vi "外观 2.vi"(0 "Data In":T9 caption="数据输入" {"数值" format="%04x"}, 2 "Display State In":T7 caption="显示状态输入" {"值" items=["三通阀", "排阀"]}, 3 "Container State":T8 caption="容器状态") -> (6 "Data Out":T9 caption="数据输出" {"数值" format="%04x"}, 7 "Display State Out":T7 caption="显示状态输出" {"值" items=["三通阀", "排阀"]}, 8 "Action":T6 caption="动作")   [LabVIEW 2016, in "CODMn调试控件V3.xctl"]
uses:
  <vilib>/_xctls/Container State.ctl
  <vilib>/_xctls/Action.ctl
  <vilib>/_xctls/XControlSupport.lvlib
panel:
  in  "缺液检测":bool caption="V2"
  in  "偏心轮:":u16 caption="mL"
  in  "模式":enum32{"测试模式", "流程模式"}(tab)
  in  "外设:":T1
  in  "加热:":bool caption="V2"
  in  "摄氏度":u16
  in  "量:":u16=5000
  in  "注射泵:":T2(radio)
  in  "进样:":T3(radio)
  out "阀配置":u8(ring) items=["三通阀", "排阀"]
  in  "柱塞泵体积/等待时间":u16=5000
  in  "功能选择":enum32{"等待", "复位", "注入", "注出"}(radio)=enum."注入"
  out "选项卡控件":enum32{"选项卡 1", "选项卡 2"}(tab)
  in  "阀口选择":T4(radio)
  in  "其他":enum32{"未选择", "更新A值", "更新B值", "反滴定"}(radio)
  in  "反应杯温度控制:":u16
  in  "偏心轮抽取液体次数:":u16
  in  "外设":T5
  out "字符串":string="柱塞泵体积μL"
  # "uL"
  # "℃"
  # "次(0代表不动作)"
  # "℃(0代表不控温)"
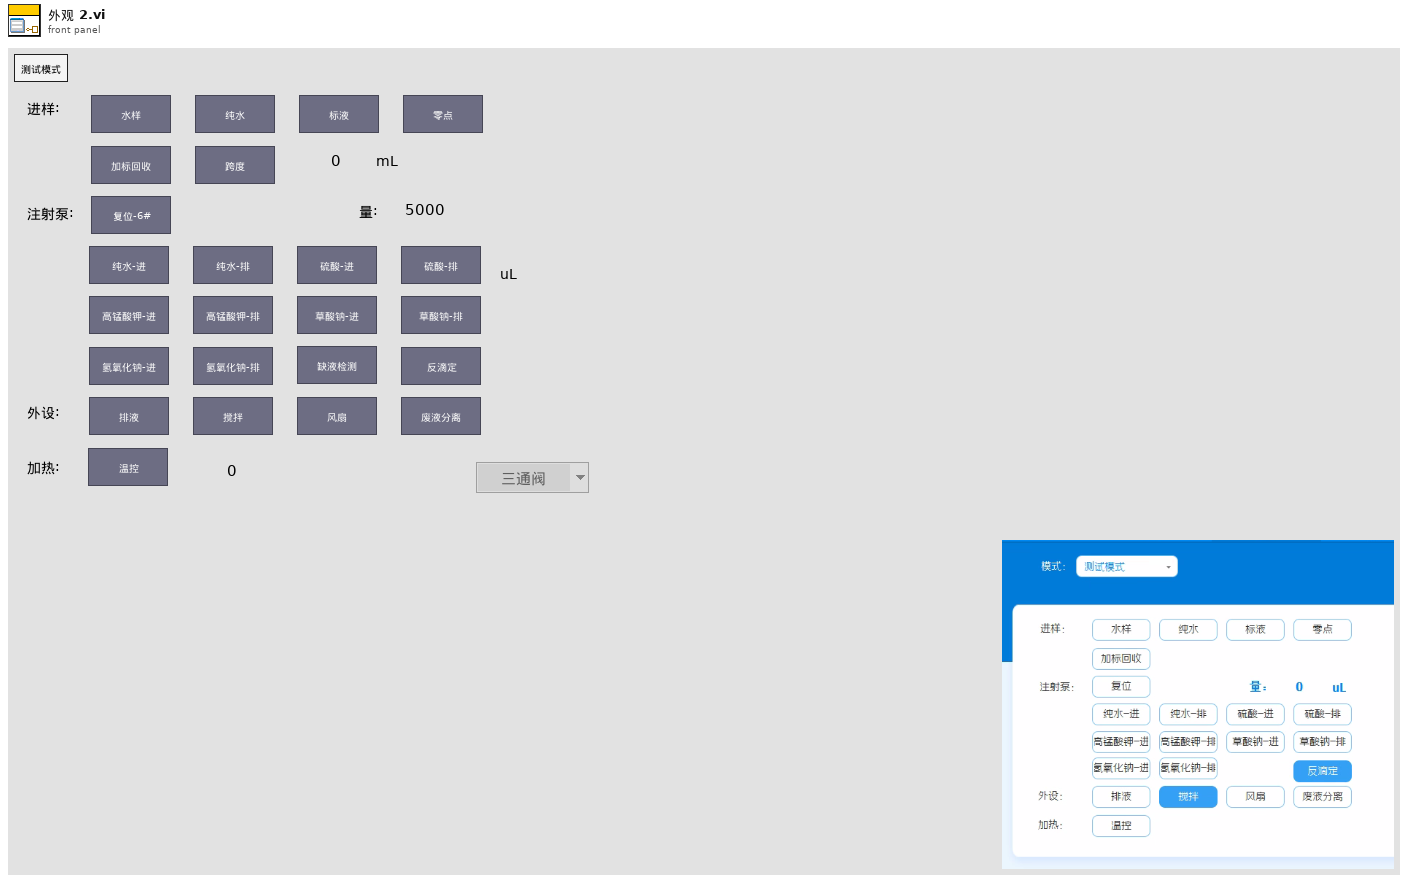
[diagram p1: front panel]
types:
  T1 = cluster{"排液":bool, "搅拌":bool, "风扇":bool, "废液分离":bool}
  T2 = enum32{"未选择", "纯水-进", "纯水-排", "硫酸-进", "硫酸-排", "复位", "高锰酸钾-进", "高锰酸钾-排", "草酸钠-进", "草酸钠-排", "氢氧化钠-进", "氢氧化钠-排", "反滴定"}
  T3 = enum32{"未选择", "水样", "纯水", "标液", "零点", "加标回收", "跨度"}
  T4 = enum32{"未选择", "V1", "V2", "V3", "V4", "V5", "V6", "V7", "V8", "V9", "V10", "V11", "V12"}
  T5 = cluster{"排液阀":bool, "搅拌":bool, "冷凝风扇":bool, "废液分离阀":bool, "电磁阀1":bool, "电磁阀2":bool, "电磁阀3":bool, "电磁阀4":bool, "电磁阀5":bool, "电磁阀6":bool}
  T6 = typedef "XControlSupport.lvlib/Action.ctl" = cluster{"Data Changed?":bool, "State Changed?":bool, "Action Name":string}
  T7 = typedef "CODMn调试控件V3.xctl/状态 2.ctl" = cluster{"值":u8}
  T8 = typedef "XControlSupport.lvlib/Container State.ctl" = cluster{"Indicator?":bool, "Run Mode?":bool, " Refnum":refnum<vi>}
  T9 = typedef "CODMn调试控件V3.xctl/数据 2.ctl" = cluster{"数值":u16[], "模式":enum32{"测试模式", "流程模式"}}
  T10 = enum32{"未选择", "水样", "纯水", "标液", "零点", "加标回收", "加标回收 2"}
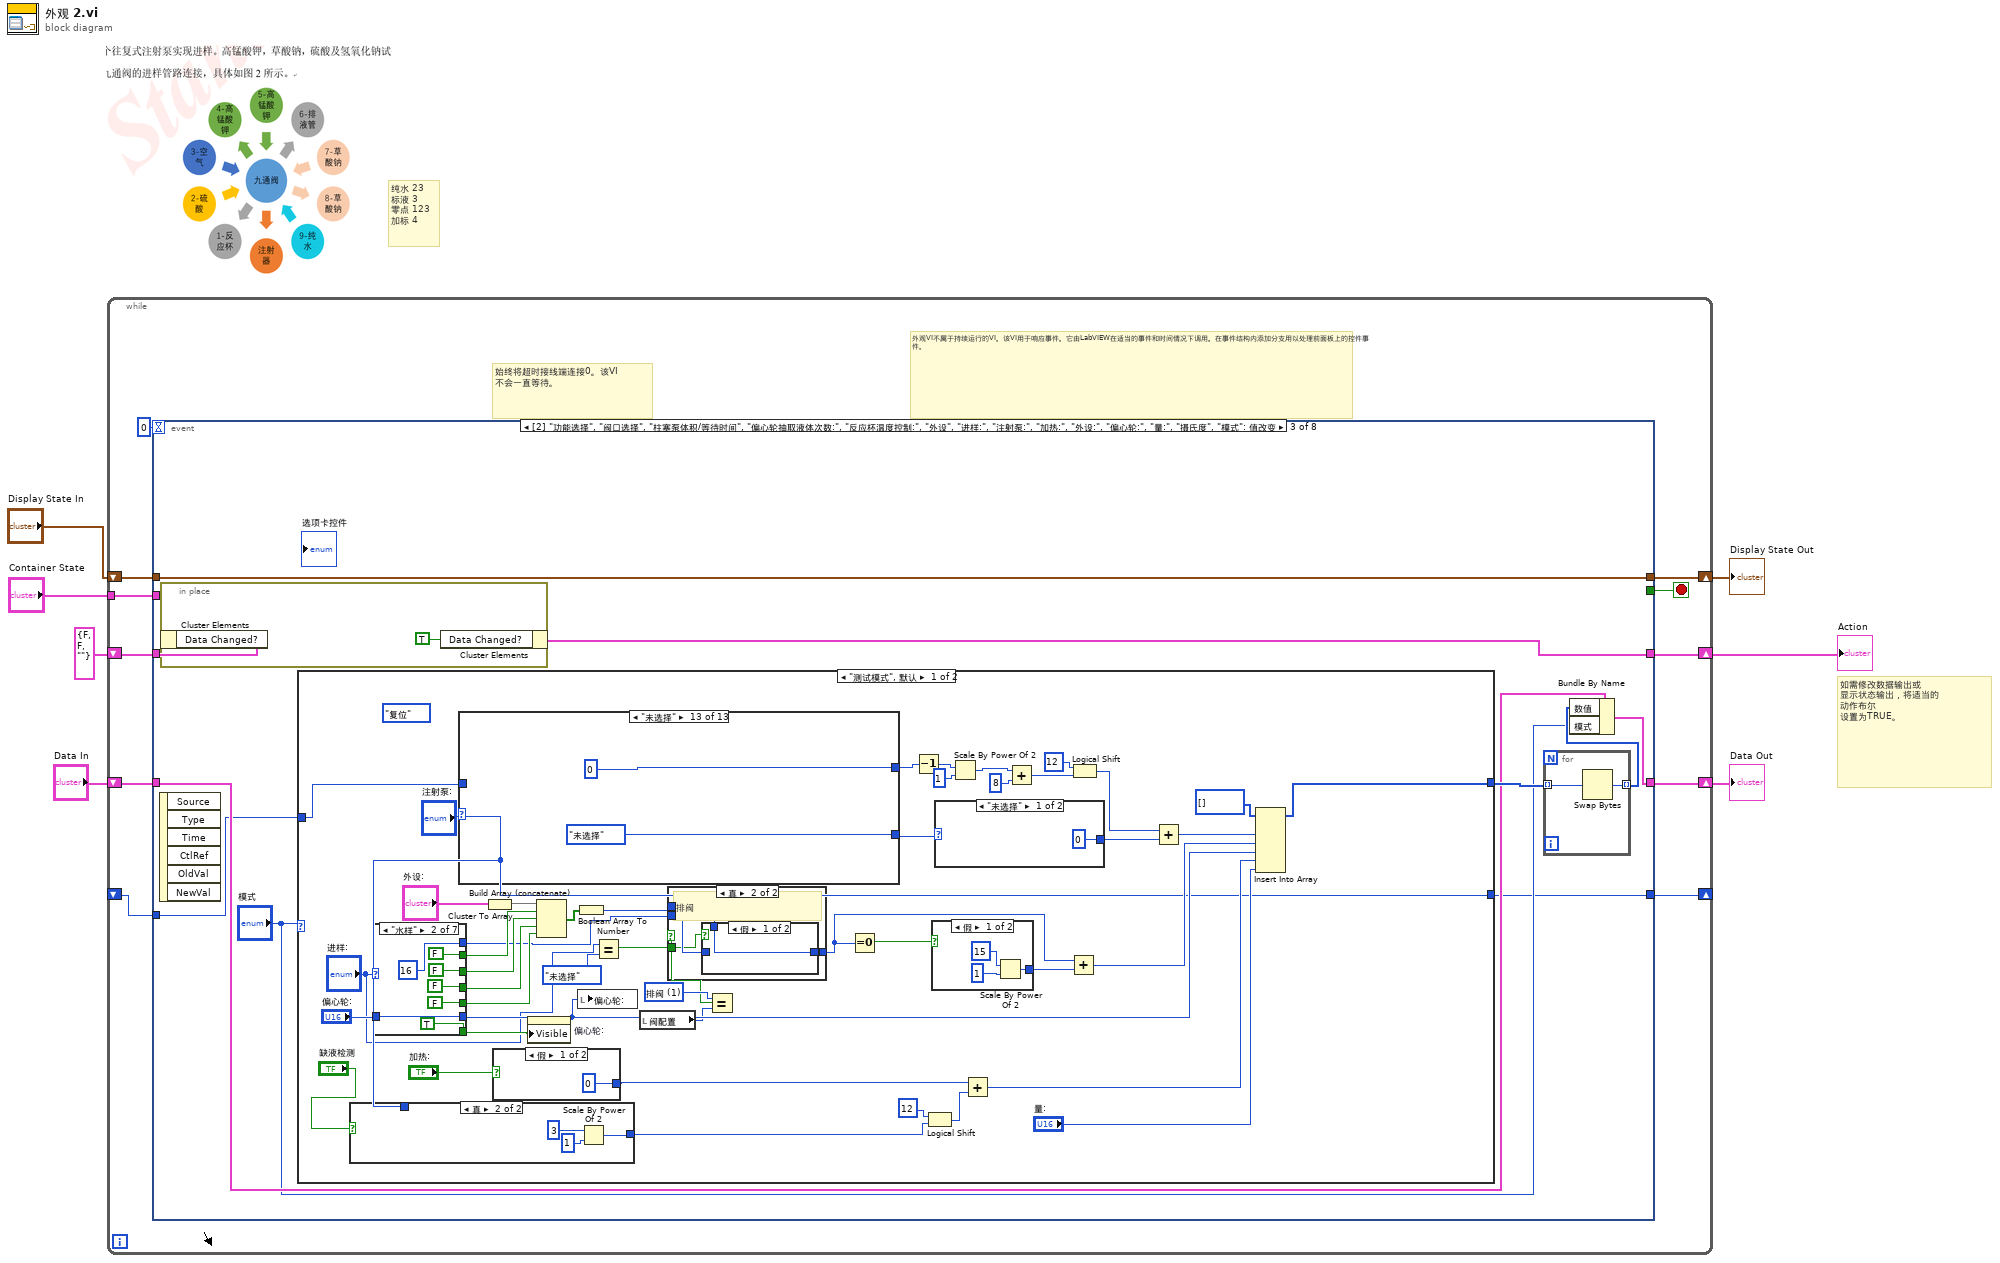
[diagram p0: block diagram]
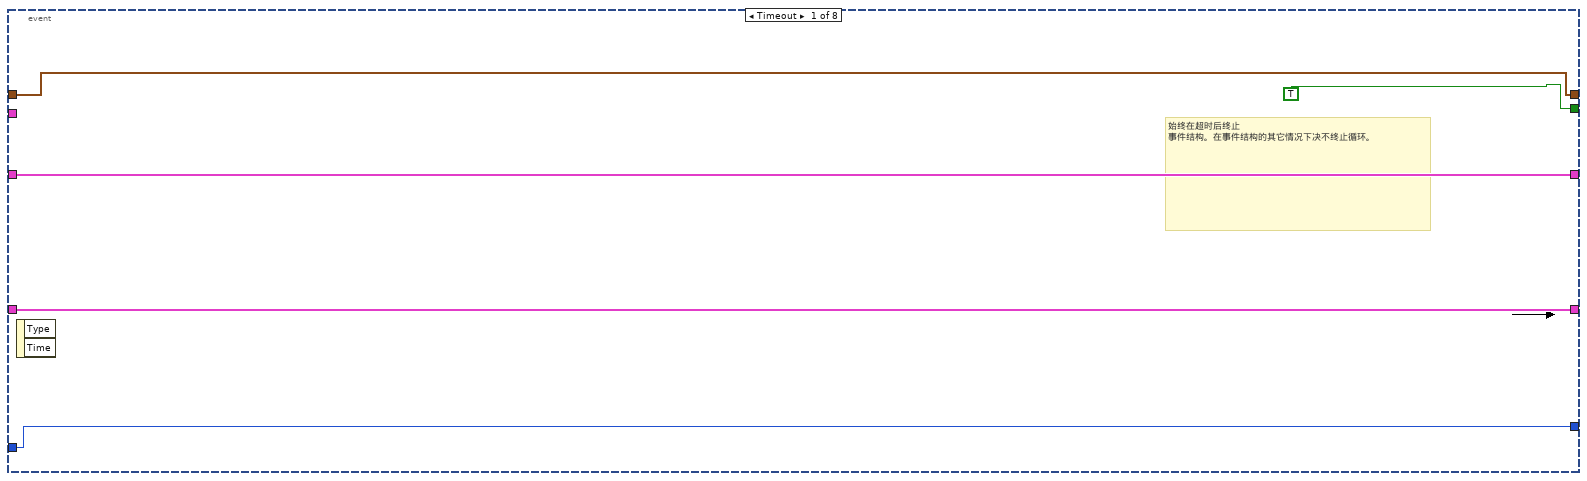
[diagram p2: hidden frame]
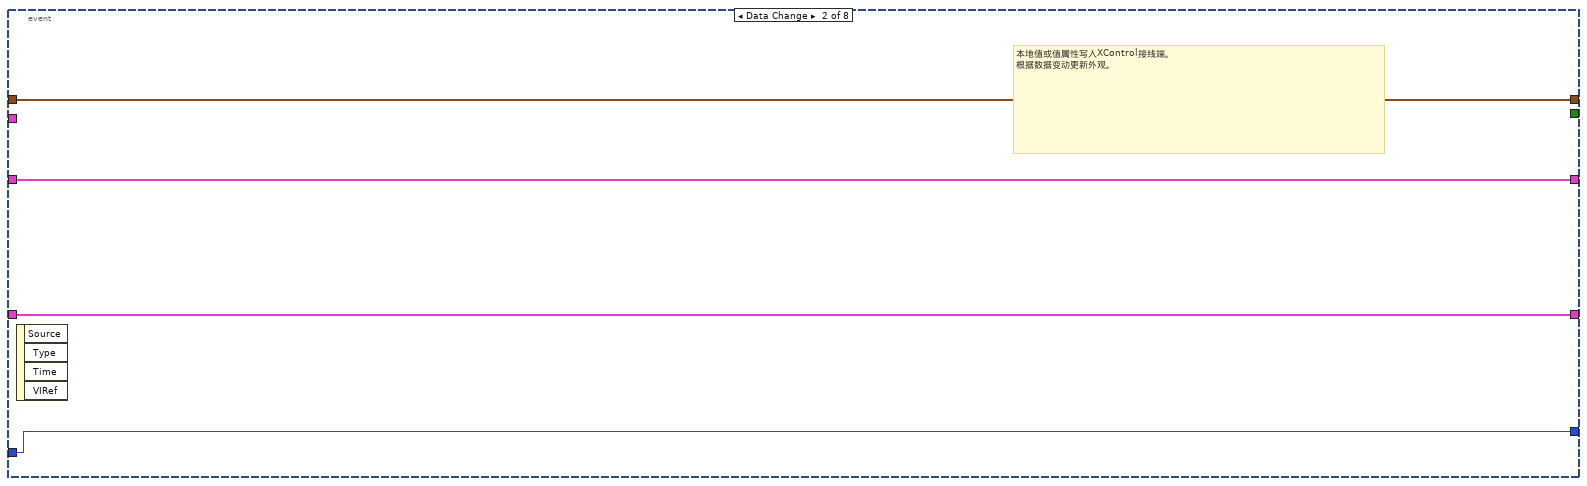
[diagram p3: hidden frame]
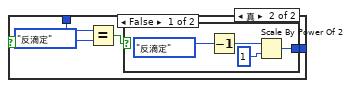
[diagram p6: hidden frame]
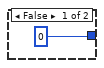
[diagram p7: hidden frame]
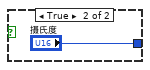
[diagram p8: hidden frame]
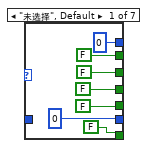
[diagram p9: hidden frame]
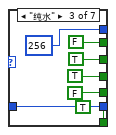
[diagram p10: hidden frame]
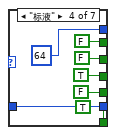
[diagram p11: hidden frame]
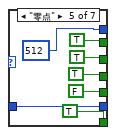
[diagram p12: hidden frame]
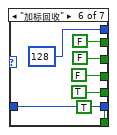
[diagram p13: hidden frame]
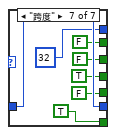
[diagram p14: hidden frame]
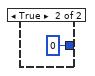
[diagram p15: hidden frame]
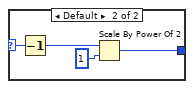
[diagram p16: hidden frame]
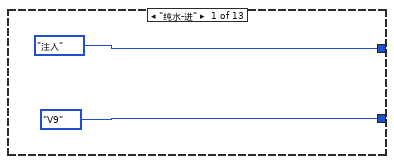
[diagram p17: hidden frame]
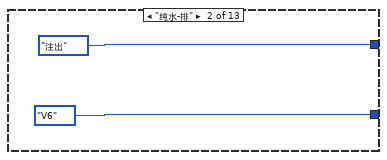
[diagram p18: hidden frame]
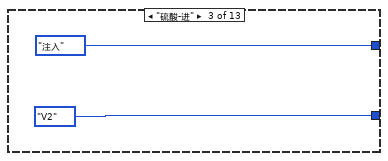
[diagram p19: hidden frame]
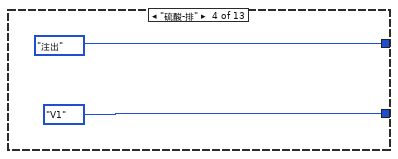
[diagram p20: hidden frame]
diagram:
  # "纯水 23\n标液 3\n零点 123\n加标 4"
  # "如需修改数据输出或\n显示状态输出，将适当的\n动作布尔\n设置为TRUE。"
  n1 = while {
    shift-right: [w17] -> w4
    shift-left: "Display State In" -> [w18]
    tunnel: "Container State" -> [w14]
    shift-right: [w12] -> w7
    shift-left: "Data In" -> [w13]
    shift-right: [w10] -> w2
    shift-left: T6 {"Data Changed?"=FALSE, "State Changed?"=FALSE, "Action Name"=""} ("Action") -> [w11]
    shift-right: [w9] -> _
    shift-left: _ -> [w8]
    stop <- w16 stop-if-true
    # "外观VI不属于持续运行的VI。该VI用于响应事件。它由LabVIEW在适当的事件和时间情况下调用。在事件结构内添加分支用以处理前面板上的控件事件。"
    # "始终将超时接线端连接0。该VI\n不会一直等待。"
    n2 = event shown="[2] \"功能选择\", \"阀口选择\", \"柱塞泵体积/等待时间\", \"偏心轮抽取液体次数:\", \"反应杯温度控制:\", \"外设\", \"进样:\", \"注射泵:\", \"加热:\", \"外设:\", \"偏心轮:\", \"量:\", \"摄氏度\", \"模式\": 值改变" {
      selector: _ -> [_ _ _ _ _ _ _ _]
      dyn-events: _ -> [_ _ _ _ _ _ _ _]
      timeout: 0 -> [_ _ _ _ _ _ _ _]
      tunnel: w18 -> [w21 w24 w37 w305 w317 w318 w326 w330]
      tunnel: [w21 w24 w37 w305 w317 w318 w326 w330] -> w17
      tunnel: [TRUE _ _ _ _ _ _ _] -> w16
      tunnel: w14 -> [_ _ _ _ _ _ w327 w332]
      tunnel: w13 -> [w20 w27 w33 w304 w316 w322 w325 w329]
      tunnel: [w20 w27 w30 w304 w316 w322 w325 w329] -> w12
      tunnel: [w22 w26 w35 w303 w315 w321 w324 w328] -> w10
      tunnel: w11 -> [w22 w26 w36 w303 w315 w321 w324 w328]
      tunnel: [w19 w25 w29 w298 w310 w320 w323 w331] -> w9
      tunnel: w8 -> [w19 w25 w28 w298 w310 w320 w323 w331]
      event Timeout {
        # "始终在超时后终止\n事件结构。在事件结构的其它情况下决不终止循环。"
        n3 = event-data() -> ()  [unwired: 1 in, 2 out]
      }
      event Data Change {
        # "本地值或值属性写入XControl接线端。\n根据数据变动更新外观。"
        n4 = event-data() -> ()  [unwired: 1 in, 4 out]
      }
      event "功能选择", "阀口选择", "柱塞泵体积/等待时间", "偏心轮抽取液体次数:", "反应杯温度控制:", "外设", "进样:", "注射泵:", "加热:", "外设:", "偏心轮:", "量:", "摄氏度", "模式": Value Change {
        n5 = event-data() -> ()  [unwired: 1 in, 6 out]
        n6 = in-place {
          n7 = in-place-cluster #1(w36) -> ()  [unwired: 1 out]
          n8 = in-place-cluster #1("Data Changed?"=TRUE) -> (w35:T6)
        }
        n9 = case shown="\"测试模式\", 默认" "模式" {
          tunnel: [w60 w249] -> w34
          tunnel: ["注射泵:" w242] -> w29
          tunnel: w28 -> [w47 w242]
          frame "测试模式", Default {
            w41 = u8 1 items=["三通阀", "排阀"] ("Value")
            (unwired) enum32{"等待", "复位", "注入", "注出"}."复位" ("功能选择")
            n10 = case shown="真" "缺液检测" {
              tunnel: "注射泵:" -> [w92 _]
              tunnel: [w90 w100] -> w62
              frame False {
                n11 = Equal?(x=w92, y=T2."反滴定" ("注射泵:")) -> (x = y?=w91:bool)
                n12 = case shown="真" w91 {
                  tunnel: [i16 0 w95] -> w90
                  frame False {
                  }
                  frame True {
                    n13 = Decrement(x=enum32{"未选择", "更新A值", "更新B值", "反滴定"}."反滴定" ("其他")) -> (x-1=w96:enum32{"未选择", "更新A值", "更新B值", "反滴定"})
                    n14 = Scale By Power Of 2(n=w96, x=i16 1 ("y")) -> (x*2^n=w95:i16)
                  }
                }
              }
              frame True {
                n15 = Scale By Power Of 2(n=i16 3, x=i16 1 ("y")) -> (x*2^n=w100:i16)
              }
            }
            n16 = case shown="\"水样\"" "进样:" {
              tunnel: [FALSE FALSE FALSE FALSE TRUE FALSE FALSE] -> w74
              tunnel: [FALSE FALSE TRUE FALSE TRUE FALSE FALSE] -> w73
              tunnel: [FALSE FALSE TRUE TRUE TRUE FALSE TRUE] -> w72
              tunnel: [FALSE FALSE FALSE FALSE FALSE TRUE FALSE] -> w71
              tunnel: "偏心轮:" -> [_ w113 w120 w127 w134 w141 w151]
              tunnel: [u16 0 ("偏心轮:") w113 w120 w127 w134 w141 w151] -> w57
              tunnel: [FALSE TRUE TRUE TRUE TRUE TRUE TRUE] -> w56
              tunnel: [u16 0 ("数字") u16 16 ("数字") u16 256 ("数字") u16 64 ("数字") u16 512 ("数字") u16 128 ("数字") u16 32 ("数字")] -> w42
              frame "未选择", Default {
              }
              frame "水样" {
              }
              frame "纯水" {
              }
              frame "标液" {
              }
              frame "零点" {
              }
              frame "加标回收" {
              }
              frame "跨度" {
              }
            }
            n17 = case shown="\"未选择\"" "注射泵:" {
              tunnel: [enum32{"等待", "复位", "注入", "注出"}."注入" ("功能选择") enum32{"等待", "复位", "注入", "注出"}."注出" ("功能选择") enum32{"等待", "复位", "注入", "注出"}."注入" ("功能选择") enum32{"等待", "复位", "注入", "注出"}."注出" ("功能选择") enum32{"等待", "复位", "注入", "注出"}."复位" ("功能选择") enum32{"等待", "复位", "注入", "注出"}."注入" ("功能选择") enum32{"等待", "复位", "注入", "注出"}."注出" ("功能选择") enum32{"等待", "复位", "注入", "注出"}."注入" ("功能选择") enum32{"等待", "复位", "注入", "注出"}."注出" ("功能选择") enum32{"等待", "复位", "注入", "注出"}."注入" ("功能选择") enum32{"等待", "复位", "注入", "注出"}."注出" ("功能选择") 0 0] -> w59
              tunnel: [T4."V9" ("阀口选择") T4."V6" ("阀口选择") T4."V2" ("阀口选择") T4."V1" ("阀口选择") T4."V6" ("阀口选择") T4."V5" ("阀口选择") T4."V4" ("阀口选择") T4."V7" ("阀口选择") T4."V8" ("阀口选择") T4."V3" ("阀口选择") T4."V6" ("阀口选择") T4."未选择" ("阀口选择") T4."未选择" ("阀口选择")] -> w80
              tunnel: w47 -> [_ _ _ _ _ w172 w181 w190 w205 w220 w229 _ _]
              frame "纯水-进" {
              }
              frame "纯水-排" {
              }
              frame "硫酸-进" {
              }
              frame "硫酸-排" {
              }
              frame "复位" {
              }
              frame "高锰酸钾-进" {
                n18 = Greater Or Equal?(x=w172, y=T2."草酸钠-进" ("注射泵:")) -> (x >= y?=w175:bool)
                n19 = Less Or Equal?(x=w172, y=T2."氢氧化钠-排" ("注射泵:")) -> (x <= y?=w176:bool)
                n20 = And(x=w175, y=w176) -> (x .and. y?=w177:bool)
                n21 = case shown="真" w177 {
                  frame False {
                  }
                  frame True {
                    n22 = One Button Dialog(message="“\"警告:未进行润洗\n或者进出液不匹配\"”" ("消息")) -> ()  [unwired: 1 in, 1 out]
                  }
                }
              }
              frame "高锰酸钾-排" {
                n23 = Greater Or Equal?(x=w181, y=T2."草酸钠-进" ("注射泵:")) -> (x >= y?=w184:bool)
                n24 = Less Or Equal?(x=w181, y=T2."氢氧化钠-排" ("注射泵:")) -> (x <= y?=w185:bool)
                n25 = And(x=w184, y=w185) -> (x .and. y?=w186:bool)
                n26 = case shown="真" w186 {
                  frame False {
                  }
                  frame True {
                    n27 = One Button Dialog(message="“\"警告:未进行润洗\n或者进出液不匹配\"”" ("消息")) -> ()  [unwired: 1 in, 1 out]
                  }
                }
              }
              frame "草酸钠-进" {
                n28 = Greater Or Equal?(x=w190, y=T2."高锰酸钾-进" ("注射泵:")) -> (x >= y?=w198:bool)
                n29 = Less Or Equal?(x=w190, y=T2."高锰酸钾-排" ("注射泵:")) -> (x <= y?=w199:bool)
                n30 = Greater Or Equal?(x=w190, y=T2."氢氧化钠-进" ("注射泵:")) -> (x >= y?=w193:bool)
                n31 = Less Or Equal?(x=w190, y=T2."氢氧化钠-排" ("注射泵:")) -> (x <= y?=w192:bool)
                n32 = And(x=w198, y=w199) -> (x .and. y?=w200:bool)
                n33 = And(x=w193, y=w192) -> (x .and. y?=w191:bool)
                n34 = Or(x=w191, y=w200) -> (x .or. y?=w201:bool)
                n35 = case shown="真" w201 {
                  frame False {
                  }
                  frame True {
                    n36 = One Button Dialog(message="“\"警告:未进行润洗\n或者进出液不匹配\"”" ("消息")) -> ()  [unwired: 1 in, 1 out]
                  }
                }
              }
              frame "草酸钠-排" {
                n37 = Greater Or Equal?(x=w205, y=T2."氢氧化钠-进" ("注射泵:")) -> (x >= y?=w208:bool)
                n38 = Less Or Equal?(x=w205, y=T2."氢氧化钠-排" ("注射泵:")) -> (x <= y?=w207:bool)
                n39 = Greater Or Equal?(x=w205, y=T2."高锰酸钾-进" ("注射泵:")) -> (x >= y?=w213:bool)
                n40 = Less Or Equal?(x=w205, y=T2."高锰酸钾-排" ("注射泵:")) -> (x <= y?=w214:bool)
                n41 = And(x=w208, y=w207) -> (x .and. y?=w206:bool)
                n42 = And(x=w213, y=w214) -> (x .and. y?=w215:bool)
                n43 = Or(x=w206, y=w215) -> (x .or. y?=w216:bool)
                n44 = case shown="真" w216 {
                  frame False {
                  }
                  frame True {
                    n45 = One Button Dialog(message="“\"警告:未进行润洗\n或者进出液不匹配\"”" ("消息")) -> ()  [unwired: 1 in, 1 out]
                  }
                }
              }
              frame "氢氧化钠-进" {
                n46 = Greater Or Equal?(x=w220, y=T2."高锰酸钾-进" ("注射泵:")) -> (x >= y?=w224:bool)
                n47 = Less Or Equal?(x=w220, y=T2."草酸钠-排" ("注射泵:")) -> (x <= y?=w225:bool)
                n48 = And(x=w224, y=w225) -> (x .and. y?=w221:bool)
                n49 = case shown="真" w221 {
                  frame False {
                  }
                  frame True {
                    n50 = One Button Dialog(message="“\"警告:未进行润洗\n或者进出液不匹配\"”" ("消息")) -> ()  [unwired: 1 in, 1 out]
                  }
                }
              }
              frame "氢氧化钠-排" {
                n51 = Greater Or Equal?(x=w229, y=T2."高锰酸钾-进" ("注射泵:")) -> (x >= y?=w233:bool)
                n52 = Less Or Equal?(x=w229, y=T2."草酸钠-排" ("注射泵:")) -> (x <= y?=w234:bool)
                n53 = And(x=w233, y=w234) -> (x .and. y?=w230:bool)
                n54 = case shown="真" w230 {
                  frame False {
                  }
                  frame True {
                    n55 = One Button Dialog(message="“\"警告:未进行润洗\n或者进出液不匹配\"”" ("消息")) -> ()  [unwired: 1 in, 1 out]
                  }
                }
              }
              frame "反滴定" {
              }
              frame "未选择" {
              }
            }
            n56 = Cluster To Array(cluster="外设:") -> (array=w75:bool[])
            n57 = case shown="假" "加热:" {
              tunnel: [u16 0 ("摄氏度") "摄氏度"] -> w63
              frame False {
              }
              frame True {
              }
            }
            n58 = property on="偏心轮:" class="DigNum (严格)"("Visible"=w56) -> ()  [unwired: 2 in, 2 out]
            n59 = Build Array (concatenate)(w75, w74, w73, w72, w71) -> (w70:bool[])
            n60 = Boolean Array To Number ("布尔数组至数值转换")(Boolean array=w70) -> (number=w44:u16)
            n61 = local write "偏心轮:"(w57) -> ()
            n62 = Equal?(x="进样:", y=T10."未选择") -> (x = y?=w39:bool)
            n63 = local read "阀配置"() -> (w40:u8)
            n64 = Equal?(x=w41, y=w40) -> (x = y?=w38:bool)
            n65 = case shown="真" w38 {
              tunnel: w44 -> [w83 w87]
              tunnel: [w83 w86] -> w43
              tunnel: w42 -> [_ w85]
              tunnel: w39 -> [_ w84]
              frame False {
              }
              frame True {
                # "排阀"
                n66 = case shown="假" w84 {
                  tunnel: w87 -> [_ w89]
                  tunnel: [w88 w89] -> w86
                  tunnel: w85 -> [w88 _]
                  frame False {
                  }
                  frame True {
                  }
                }
              }
            }
            n67 = Equal To 0?(x=w43) -> (x = 0?=w77:bool)
            n68 = Decrement(x=w59) -> (x-1=w50:u32)
            n69 = Logical Shift(y=i16 12, x=w62) -> (x << y=w64:i16)
            n70 = case shown="假" w77 {
              tunnel: [w153 u16 0] -> w78
              frame False {
                n71 = Scale By Power Of 2(n=i16 15, x=u16 1 ("y")) -> (x*2^n=w153:u16)
              }
              frame True {
              }
            }
            n72 = case shown="\"未选择\"" w80 {
              selector: w80 -> [_ w159]
              tunnel: [i16 0 ("y") w161] -> w82
              frame "未选择" {
              }
              frame Default {
                n73 = Decrement(x=w159) -> (x-1=w160:T4)
                n74 = Scale By Power Of 2(n=w160, x=i16 1 ("y")) -> (x*2^n=w161:i16)
              }
            }
            n75 = Scale By Power Of 2(n=w50, x=i16 1 ("y")) -> (x*2^n=w53:i16)
            n76 = Add(x=w63, y=w64) -> (x+y=w61:u16)
            n77 = Add(x=w53, y=i16 8) -> (x+y=w54:i16)
            n78 = Add(x=w43, y=w78) -> (x+y=w68:u16)
            n79 = Logical Shift(y=i16 12, x=w54) -> (x << y=w81:i16)
            n80 = Add(x=w81, y=w82) -> (x+y=w69:i16)
            n81 = Insert Into Array(array=u16[] [] ("数组"), new element #1=w69, new element #2=w68, new element #3=w57, new element #4=w61, new element #5="量:") -> (w60:u16[])  [unwired: 1 in]
          }
          frame "流程模式" {
            n82 = case shown="\"等待\"" "功能选择" {
              selector: "功能选择" -> [_ w283]
              tunnel: [enum32{"选项卡 1", "选项卡 2"}."选项卡 2" ("选项卡控件") enum32{"选项卡 1", "选项卡 2"}."选项卡 1" ("选项卡控件")] -> w255
              tunnel: [w266 u16 0] -> w248
              tunnel: [i16 0 ("y") w284] -> w243
              frame "等待" {
                n83 = Cluster To Array(cluster="外设") -> (array=w267:bool[])
                n84 = Boolean Array To Number ("布尔数组至数值转换")(Boolean array=w267) -> (number=w270:u16)
                n85 = Equal To 0?(x=w270) -> (x = 0?=w269:bool)
                n86 = case shown="假" w269 {
                  tunnel: [w273 u16 0] -> w271
                  frame False {
                    n87 = Scale By Power Of 2(n=i16 15, x=u16 1 ("y")) -> (x*2^n=w273:u16)
                  }
                  frame True {
                  }
                }
                n88 = Add(x=w270, y=w271) -> (x+y=w266:u16)
              }
              frame Default {
                n89 = Decrement(x=w283) -> (x-1=w277:enum32{"等待", "复位", "注入", "注出"})
                n90 = case shown="默认" "阀口选择" {
                  selector: "阀口选择" -> [_ w292]
                  tunnel: [i16 0 ("y") w294] -> w285
                  frame "未选择" {
                  }
                  frame Default {
                    n91 = Decrement(x=w292) -> (x-1=w293:T4)
                    n92 = Scale By Power Of 2(n=w293, x=i16 1 ("y")) -> (x*2^n=w294:i16)
                  }
                }
                n93 = Scale By Power Of 2(n=w277, x=i16 1 ("y")) -> (x*2^n=w280:i16)
                n94 = Add(x=w280, y=i16 8) -> (x+y=w279:i16)
                n95 = Logical Shift(y=i16 12, x=w279) -> (x << y=w286:i16)
                n96 = Add(x=w286, y=w285) -> (x+y=w284:i16)
              }
            }
            n97 = case shown="\"未选择\"" "其他" {
              tunnel: "其他" -> [_ w261]
              tunnel: [i16 0 w260] -> w246
              frame "未选择" {
              }
              frame "更新A值", Default {
                n98 = Decrement(x=w261) -> (x-1=w263:enum32{"未选择", "更新A值", "更新B值", "反滴定"})
                n99 = Scale By Power Of 2(n=w263, x=i16 1 ("y")) -> (x*2^n=w260:i16)
              }
            }
            n100 = Logical Shift(y=i16 12, x=w246) -> (x << y=w245:i16)
            n101 = feedback #2() -> (w257:enum32{"选项卡 1", "选项卡 2"})  [unwired: 1 in]
            n102 = feedback-in #2(w255) -> ()
            n103 = Add(x="反应杯温度控制:", y=w245) -> (x+y=w250:u16)
            n104 = Not Equal?(x=w255, y=w257) -> (x != y?=w256:bool)
            n105 = case shown="真" w256 {
              tunnel: w255 -> [_ w264]
              frame False {
              }
              frame True {
                n106 = property on="选项卡控件" class="TabCtl (严格)"("Val(Sgnl)"=w264) -> ()  [unwired: 2 in, 2 out]
              }
            }
            n107 = Insert Into Array(array=u16[] [] ("数组"), new element #1=w243, new element #2=w248, new element #3="偏心轮抽取液体次数:", new element #4=w250, new element #5="柱塞泵体积/等待时间") -> (w249:u16[])  [unwired: 1 in]
          }
        }
        n108 = for {
          tunnel: w34 -> [w296] mode=indexing
          tunnel: [w295] -> w32 mode=indexing
          n109 = Swap Bytes(anything=w296) -> (byte swapped=w295:u16)
        }
        n110 = Bundle By Name(cluster=w33, "数值"=w32, "模式"="模式") -> (w30:T9)
      }
      event "选项卡控件": Value Change {
        n111 = event-data() -> ("NewVal"=w302:enum32{"选项卡 1", "选项卡 2"})  [unwired: 1 in, 5 out]
        n112 = case shown="\"选项卡 1\", 默认" w302 {
          tunnel: [i16 5000 ("数值") i16 60 ("数值")] -> w301
          tunnel: ["柱塞泵体积μL" ("字符串") "等待时间秒" ("字符串")] -> w299
          frame "选项卡 1", Default {
          }
          frame "选项卡 2" {
          }
        }
        "字符串" <- w299
        n113 = local write "阀口选择"(T4."未选择" ("阀口选择")) -> ()
        n114 = local write "柱塞泵体积/等待时间"(w301) -> ()
      }
      event "柱塞泵体积/等待时间", "偏心轮抽取液体次数:", "反应杯温度控制:", "偏心轮:", "量:", "摄氏度": Mouse Down {
        n115 = event-data() -> ("CtlRef"=w314:refnum<vi>)  [unwired: 1 in, 7 out]
        n116 = property class="DigNum (严格)"(reference=w314) -> (reference out=w313:refnum<vi>, "Value"=w312:u16)  [unwired: 1 in, 1 out]
        n117 = call "数字键盘.vi"("OldNumber"=w312) -> ("NewNumber"=w311:sgl)
        n118 = property class="DigNum (严格)"(reference=w313, "Val(Sgnl)"=w311) -> ()  [unwired: 1 in, 2 out]
      }
      event Display State Change {
        # "拖放该XControl的新实例、复制、撤消操作或者在XControl内执行自定义属性或方法均可改变显示状态。更新相应外观。"
        n119 = event-data() -> ()  [unwired: 1 in, 4 out]
        n120 = Unbundle By Name(w318) -> ("值"=→"阀配置":u8)
      }
      event Direction Change {
        # "XControl的方向由输入控件转换为显示控件，反之亦然。更新相应外观。"
        n121 = event-data() -> ()  [unwired: 1 in, 4 out]
        n122 = Unbundle By Name(w327) -> ()  [unwired: 1 out]
      }
      event Exec State Change {
        # "包含该XControl的VI已从编辑模式切换至运行模式，反之亦然。\n相应的更新外观。"
        # "分别处理编辑模式和\n运行模式"
        n123 = event-data() -> ()  [unwired: 1 in, 4 out]
        n124 = Unbundle By Name(w332) -> ()  [unwired: 1 out]
      }
    }
  }
  "Display State Out" <- w4
  "Data Out" <- w7
  "Action" <- w2
